vi "Square Inputs.vi"(7 "Square Input":bool=TRUE, 11 "Joystick Input":dbl) -> (3 "Joystick Output":dbl)   [LabVIEW 2017]
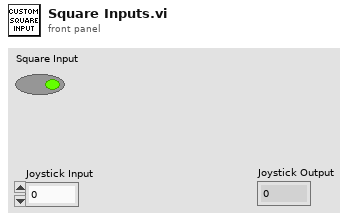
[diagram p1: front panel]
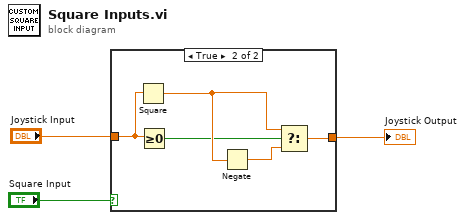
[diagram p0: block diagram]
diagram:
  n1 = case shown="True" "Square Input" {
    tunnel: [w4 w9] -> w1
    tunnel: "Joystick Input" -> [w4 w8]
    frame False {
    }
    frame True {
      n2 = Square(x=w8) -> (x^2=w6:dbl)
      n3 = Greater Or Equal To 0?(x=w8) -> (x >= 0?=w5:bool)
      n4 = Negate(x=w6) -> (-x=w7:dbl)
      n5 = Select(t=w6, s=w5, f=w7) -> (s? t:f=w9:dbl)
    }
  }
  "Joystick Output" <- w1
